vi "Group.Find.vi"(8 "error in (no error)":errorcluster, 9 "Name":string, 11 "Parent":T1 format="%.0x") -> (0 "error out":errorcluster, 1 "Child Name":string, 2 "Child":T1 format="%.0x", 3 "Parent":T1 format="%.0x")   [LabVIEW 2019, in "Fuel Injector Analysis Addon System Explorer.lvlib"]
uses:
  Fuel Injector Analysis Addon System Explorer.lvlib
  <vilib>/NI VeriStand/Custom Device API/Custom Device Item Ref.ctl
  Addon Shared/SubVIs/Constants.vi
  <vilib>/NI VeriStand/Custom Device Tools/Custom Device Utility Library/NI VeriStand - Search for All Items by GUID.vi
  <vilib>/NI VeriStand/Custom Device Tools/Custom Device Utility Library/Custom Device Utility Library.lvlib
  <vilib>/NI VeriStand/Custom Device Tools/Custom Device Utility Library/NI VeriStand - Search for Item by Name.vi
  Addon Shared/Fuel Injector Analysis Addon Shared.lvlib
  <vilib>/NI VeriStand/Custom Device API/Custom Device API.lvlib
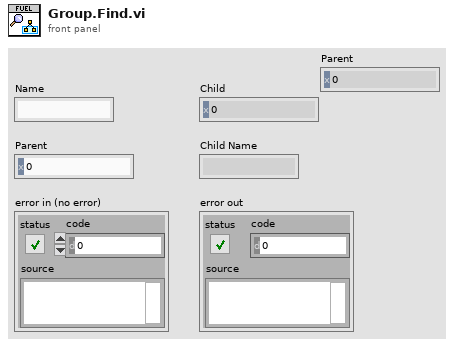
[diagram p1: front panel]
types:
  T1 = typedef "Custom Device API.lvlib/Custom Device Item Ref.ctl" = u64
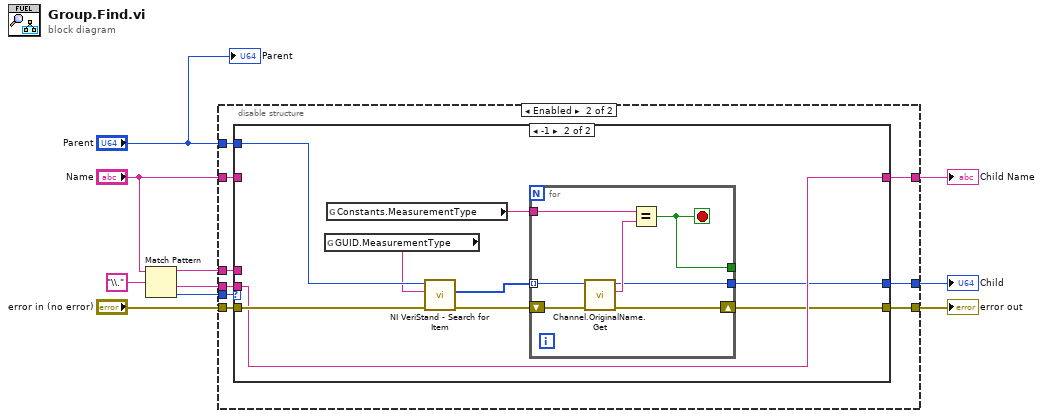
[diagram p0: block diagram]
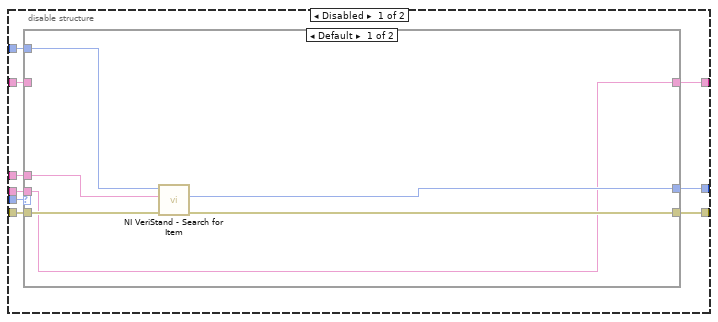
[diagram p2: hidden frame]
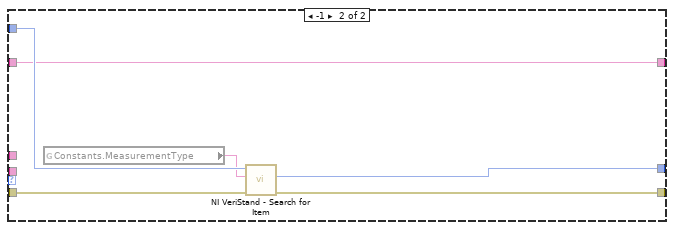
[diagram p3: hidden frame]
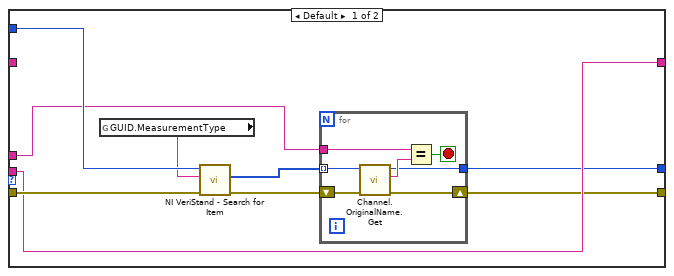
[diagram p4: hidden frame]
diagram:
  n1 = Match Pattern(string="Name", regular expression="\\.") -> (before substring=w4:string, after substring=w10:string, offset past match=w2:i32)  [unwired: 1 in, 1 out]
  n2 = disable-structure shown="Enabled" {
    disable-tunnel: w10 -> [w19 w40]
    disable-tunnel: "Name" -> [w18 w39]
    disable-tunnel: [w17 w38] -> w8
    disable-tunnel: [w16 w37] -> w7
    disable-tunnel: "Parent" -> [w15 w36]
    disable-tunnel: [w14 w35] -> w5
    disable-tunnel: w4 -> [w13 w34]
    disable-tunnel: "error in (no error)" -> [w12 w33]
    disable-tunnel: w2 -> [w11 w32]
    frame Disabled {
      n3 = case shown="Default" w11 {
        tunnel: w12 -> [w25 w31]
        tunnel: w13 -> [w21 _]
        tunnel: w15 -> [w24 w28]
        tunnel: [w23 w30] -> w14
        tunnel: [w22 w29] -> w16
        tunnel: [w20 w26] -> w17
        tunnel: w18 -> [_ w26]
        tunnel: w19 -> [w20 _]
        frame Default {
          n4 = call-poly <vilib>:"NI VeriStand - Search for Item.vi"("error in"=w25, "Item Name"=w21, "Section Ref in"=w24) -> ("error out"=w23:errorcluster, "Item Ref"=w22:T1)  [unwired: 5 in, 2 out]
        }
        frame -1 {
          n5 = global read "Constants.vi" "Constants.MeasurementType"() -> (w27:string)
          n6 = call-poly <vilib>:"NI VeriStand - Search for Item.vi"("error in"=w31, "Item Name"=w27, "Section Ref in"=w28) -> ("error out"=w30:errorcluster, "Item Ref"=w29:T1)  [unwired: 5 in, 2 out]
        }
      }
    }
    frame Enabled {
      n7 = case shown="-1" w32 {
        tunnel: w33 -> [w49 w65]
        tunnel: w34 -> [w42 _]
        tunnel: w36 -> [w47 w63]
        tunnel: [w44 w60] -> w35
        tunnel: [w41 w58] -> w37
        tunnel: [w48 w64] -> w38
        tunnel: w39 -> [_ _]
        tunnel: w40 -> [w48 w64]
        frame Default {
          n8 = global read "Constants.vi" "GUID.MeasurementType"() -> (w46:string)
          n9 = call-poly <vilib>:"NI VeriStand - Search for Item.vi"("error in"=w49, "Item GUID"=w46, "Section Ref in"=w47) -> ("error out"=w45:errorcluster, "Item Refs"=w43:T1[])  [unwired: 5 in, 2 out]
          n10 = for {
            shift-right: [w55] -> w44
            shift-left: w45 -> [w56]
            tunnel: w43 -> [w54] mode=indexing
            tunnel: w42 -> [w52]
            tunnel: [w50] -> w41
            stop <- w51 stop-if-true
            n11 = call "Channel.OriginalName.Get.vi"("error in (no error)"=w56, "Ref in"=w54) -> ("error out"=w55:errorcluster, "Value"=w53:string, "Ref out"=w50:T1)  [unwired: 6 in, 1 out]
            n12 = Equal?(x=w52, y=w53) -> (x = y?=w51:bool)
          }
        }
        frame -1 {
          n13 = global read "Constants.vi" "GUID.MeasurementType"() -> (w62:string)
          n14 = global read "Constants.vi" "Constants.MeasurementType"() -> (w57:string)
          n15 = call-poly <vilib>:"NI VeriStand - Search for Item.vi"("error in"=w65, "Item GUID"=w62, "Section Ref in"=w63) -> ("error out"=w61:errorcluster, "Item Refs"=w59:T1[])  [unwired: 5 in, 2 out]
          n16 = for {
            shift-right: [w71] -> w60
            shift-left: w61 -> [w72]
            tunnel: w59 -> [w70] mode=indexing
            tunnel: w57 -> [w68]
            tunnel: [w67] -> w58
            tunnel: [w66] -> _
            stop <- w66 stop-if-true
            n17 = call "Channel.OriginalName.Get.vi"("error in (no error)"=w72, "Ref in"=w70) -> ("error out"=w71:errorcluster, "Value"=w69:string, "Ref out"=w67:T1)  [unwired: 6 in, 1 out]
            n18 = Equal?(x=w68, y=w69) -> (x = y?=w66:bool)
          }
        }
      }
    }
  }
  "Child Name" <- w8
  "Child" <- w7
  "error out" <- w5
  "Parent" <- "Parent"
